vi "Largest Buffer Size (Transfer Group).vi"(8 "error in (no error)":errorcluster, 9 "prev engine buffer size (0)":u64 format="%d bytes", 10 "prev string buffer size (0)":u64 format="%d bytes", 11 "Transfer Group Configuration in":T1={"name"="", "direction"=enum."Tx", "cycle timing"={"priority"=0, "decimation"=1, "offset"=0}, "thread index"=-1, "settings"=[], "Transfers"=[], "timeout behavior"=enum."Increment Late Count"} {"Transfers"."channels"."string offset" format="%d bytes"}) -> (0 "error out":errorcluster, 1 "largest engine buffer size":u64 format="%d bytes", 2 "largest string buffer size":u64 format="%d bytes", 3 "Transfer Group Configuration out":T1={"name"="", "direction"=enum."Tx", "cycle timing"={"priority"=0, "decimation"=1, "offset"=0}, "thread index"=-1, "settings"=[], "Transfers"=[], "timeout behavior"=enum."Increment Late Count"} {"Transfers"."channels"."string offset" format="%d bytes"})   [LabVIEW 2017, in "DSF Core.lvlib"]
uses:
  DSF Core.lvlib
  Controls/DSF Engine Transfer Group Configuration.ctl
  Controls/DSF Direction.ctl
  Controls/DSF Timing Info.ctl
  Controls/DSF Settings Info.ctl
  Controls/DSF Engine Transfer Configuration.ctl
  Controls/DSF Byte Order.ctl
  Controls/DSF Engine Channel Configuration.ctl
  Controls/DSF Data Type.ctl
  Controls/DSF Timeout Behavior.ctl
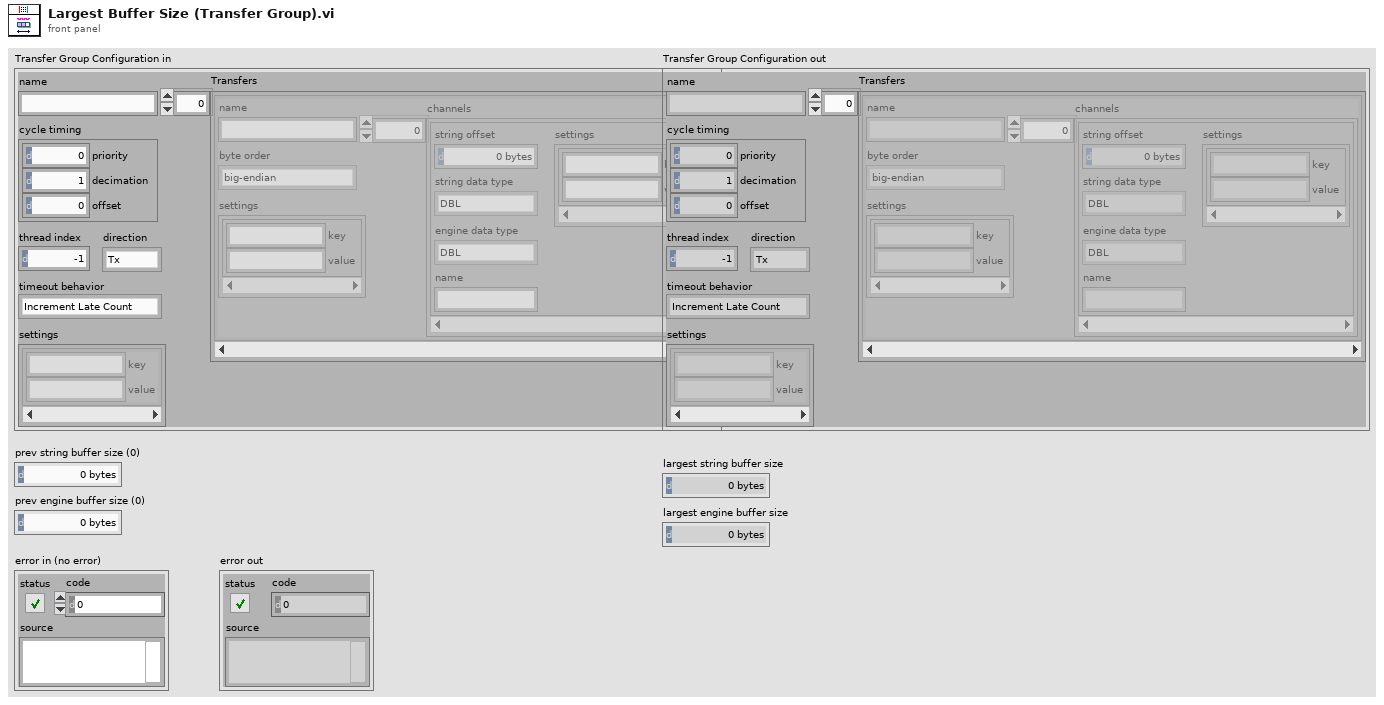
[diagram p1: front panel]
types:
  T1 = typedef "DSF Core.lvlib/DSF Engine Transfer Group Configuration.ctl" = cluster{"name":string, "direction":T2, "cycle timing":T3, "thread index":i32, "settings":T4, "Transfers":T5[], "timeout behavior":T9}
  T2 = typedef "DSF Core.lvlib/DSF Direction.ctl" = enum8{"Tx", "Rx"}
  T3 = typedef "DSF Core.lvlib/DSF Timing Info.ctl" = cluster{"priority":u64, "decimation":u64, "offset":u64}
  T4 = typedef "DSF Core.lvlib/DSF Settings Info.ctl" = cluster{"key":string, "value":string}[]
  T5 = typedef "DSF Core.lvlib/DSF Engine Transfer Configuration.ctl" = cluster{"name":string, "byte order":T6, "settings":T4, "channels":T7[]}
  T6 = typedef "DSF Core.lvlib/DSF Byte Order.ctl" = enum8{"big-endian", "little-endian"}
  T7 = typedef "DSF Core.lvlib/DSF Engine Channel Configuration.ctl" = cluster{"string offset":u64, "string data type":T8, "engine data type":T8, "name":string, "settings":T4}
  T8 = typedef "DSF Core.lvlib/DSF Data Type.ctl" = enum8{"Bool", "SGL", "DBL", "I8", "I16", "I32", "I64", "U8", "U16", "U32", "U64"}
  T9 = typedef "DSF Core.lvlib/DSF Timeout Behavior.ctl" = enum8{"Increment Late Count", "Throw Error"}
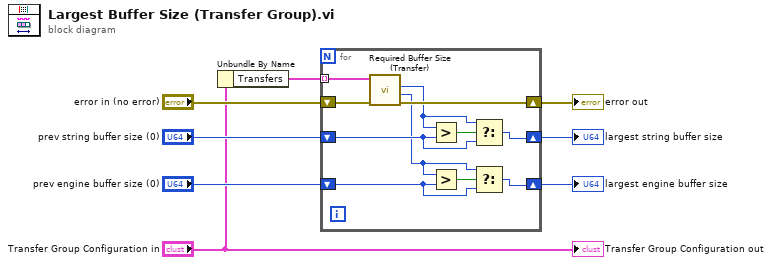
[diagram p0: block diagram]
diagram:
  n1 = Unbundle By Name("Transfer Group Configuration in") -> ("Transfers"=w7:T5[])
  n2 = for {
    tunnel: w7 -> [w19] mode=indexing
    shift-right: [w15] -> w8
    shift-left: "prev string buffer size (0)" -> [w14]
    shift-right: [w18] -> w5
    shift-left: "error in (no error)" -> [w17]
    shift-right: [w9] -> w4
    shift-left: "prev engine buffer size (0)" -> [w11]
    n3 = call "Required Buffer Size (Transfer).vi"("error in (no error)"=w17, "Transfer Configuration in"=w19) -> ("error out"=w18:errorcluster, "engine buffer size"=w10:u64, "string buffer size"=w13:u64)  [unwired: 6 in, 1 out]
    n4 = Greater?(x=w13, y=w14) -> (0:w16:bool)
    n5 = Greater?(x=w10, y=w11) -> (0:w12:bool)
    n6 = Select(t=w13, s=w16, f=w14) -> (s? t:f=w15:u64)
    n7 = Select(t=w10, s=w12, f=w11) -> (s? t:f=w9:u64)
  }
  "largest string buffer size" <- w8
  "error out" <- w5
  "largest engine buffer size" <- w4
  "Transfer Group Configuration out" <- "Transfer Group Configuration in"
